vi "Onenote_Auth_handler.vi"(8 "error in (no error)":errorcluster, 10 "Auth Time In":dbl, 11 "Paths":T2) -> (0 "error out":errorcluster, 2 "Auth Time Out":dbl, 3 "Codes":T1)   [LabVIEW 2016]
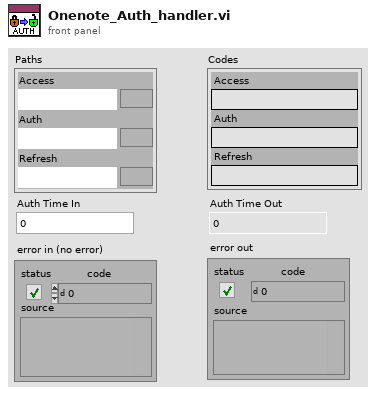
[diagram p1: front panel]
types:
  T1 = cluster{"Access":string, "Auth":string, "Refresh":string}
  T2 = cluster{"Access":path, "Auth":path, "Refresh":path}
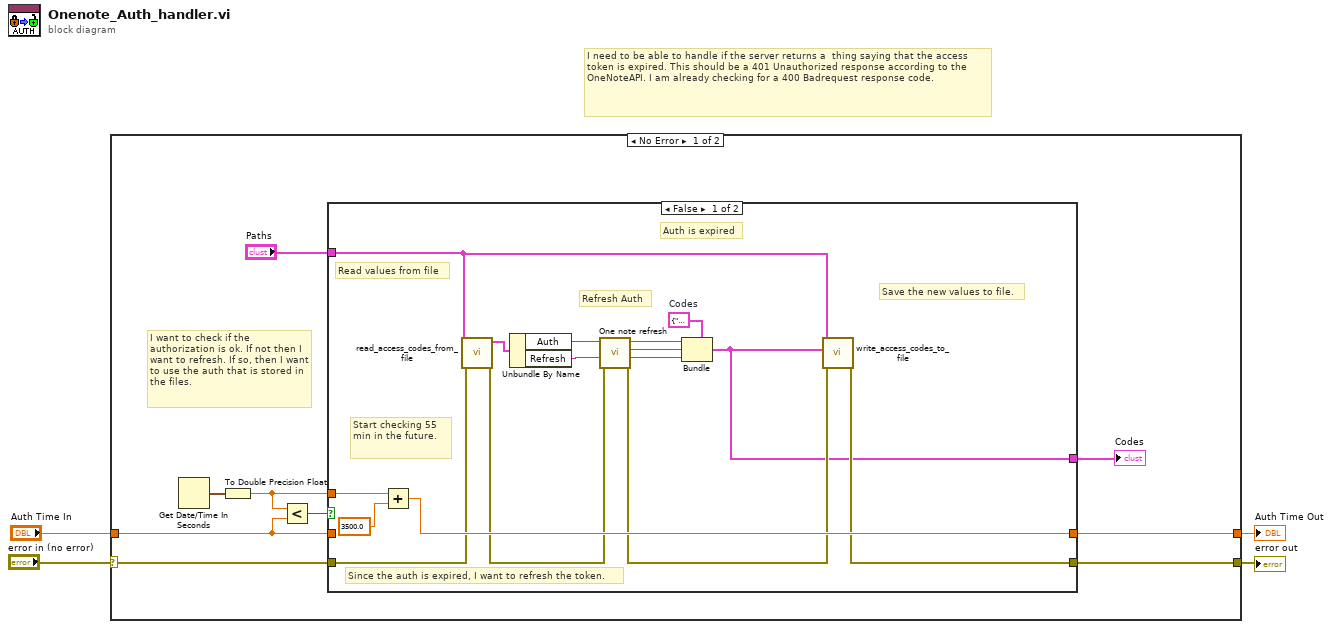
[diagram p0: block diagram]
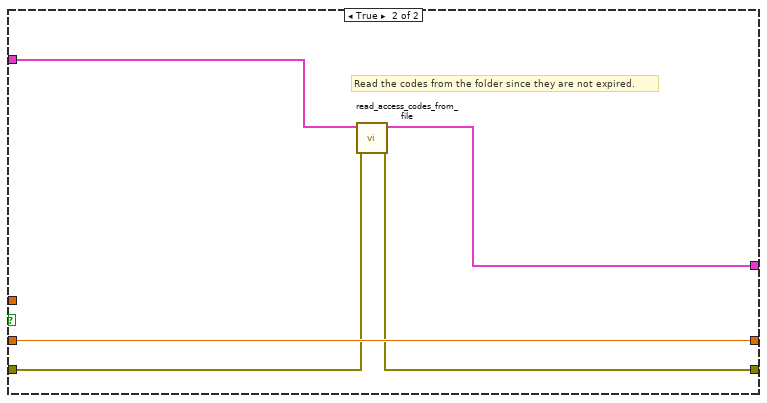
[diagram p2: hidden frame]
diagram:
  # "I need to be able to handle if the server returns a  thing saying that the access token is expired. This should be a 401 Unauthorized response according to the OneNoteAPI. I am already checking for a 400 Badrequest response code."
  n1 = case shown="No Error" "error in (no error)" {
    selector: "error in (no error)" -> [w9 w36]
    tunnel: [w8 w36] -> w3
    tunnel: "Auth Time In" -> [w7 w35]
    tunnel: [w6 w35] -> w1
    frame No Error {
      # "I want to check if the authorization is ok. If not then I want to refresh. If so, then I want to use the auth that is stored in the files."
      n2 = Get Date/Time In Seconds() -> (seconds since 1Jan1904=w13:timestamp)
      n3 = To Double Precision Float(number=w13) -> (double precision float=w11:dbl)
      n4 = Less?(x=w11, y=w7) -> (x < y?=w12:bool)
      n5 = case shown="False" w12 {
        tunnel: w7 -> [_ w34]
        tunnel: w11 -> [w29 _]
        tunnel: [w27 w34] -> w6
        tunnel: "Paths" -> [w19 w33]
        tunnel: w9 -> [w17 w30]
        tunnel: [w21 w32] -> w8
        tunnel: [w20 w31] -> w5
        frame False {
          w26 = T1 {"Access"="", "Auth"="", "Refresh"=""}  # Codes
          # "Start checking 55 min in the future."
          # "Refresh Auth"
          # "Read values from file"
          # "Save the new values to file."
          # "Auth is expired"
          # "Since the auth is expired, I want to refresh the token."
          n6 = Add(x=w29, y=3500.0) -> (x+y=w27:dbl)
          n7 = call "read_access_codes_from_file.vi"("error in (no error)"=w17, "Paths"=w19) -> ("error out"=w16:errorcluster, "Codes"=w18:T1)  [unwired: 8 in]
          n8 = Unbundle By Name(w18) -> ("Auth"=w14:string, "Refresh"=w15:string)
          n9 = call "One note refresh.vi"("error in"=w16, "Refresh Token In"=w15, "Authorization Code In"=w14) -> ("error out"=w22:errorcluster, "Refresh Token Out"=w23:string, "Access Token Out"=w24:string, "Auth Code Out"=w25:string)  [unwired: 5 in]
          n10 = Bundle(cluster=w26, "Access"=w25, "Auth"=w24, "Refresh"=w23) -> (w20:T1)
          n11 = call "write_access_codes_to_file.vi"("error in"=w22, "Codes"=w20, "Paths In"=w19) -> ("error out"=w21:errorcluster)  [unwired: 8 in]
        }
        frame True {
          # "Read the codes from the folder since they are not expired."
          n12 = call "read_access_codes_from_file.vi"("error in (no error)"=w30, "Paths"=w33) -> ("error out"=w32:errorcluster, "Codes"=w31:T1)  [unwired: 8 in]
        }
      }
      "Codes" <- w5
    }
    frame Error {
    }
  }
  "error out" <- w3
  "Auth Time Out" <- w1
